vi "ReadLeftShiftRegister.vi"(1 "reference":refnum<vi>) -> (0 "LeftShiftRegister":T4)   [LabVIEW 2013]
uses:
  <vilib>/Utility/miscctls.llb/LVBoundsTypeDef.ctl
  <vilib>/Utility/miscctls.llb/LVPositionTypeDef.ctl
  <vilib>/Utility/miscctls.llb/LVRectTypeDef.ctl
panel:
  out "error out 17":errorcluster
  out "error out 16":errorcluster
  out "error out 15":errorcluster
  out "error out 14":errorcluster
  out "error out 13":errorcluster
  out "error out 12":errorcluster
  out "error out 11":errorcluster
  out "error out 10":errorcluster
  out "error out 9":errorcluster
  out "error out 8":errorcluster
  out "error out 7":errorcluster
  out "error out 6":errorcluster
  out "error out 5":errorcluster
  out "error out 4":errorcluster
  out "error out 3":errorcluster
  out "error out 2":errorcluster
  out "error out":errorcluster
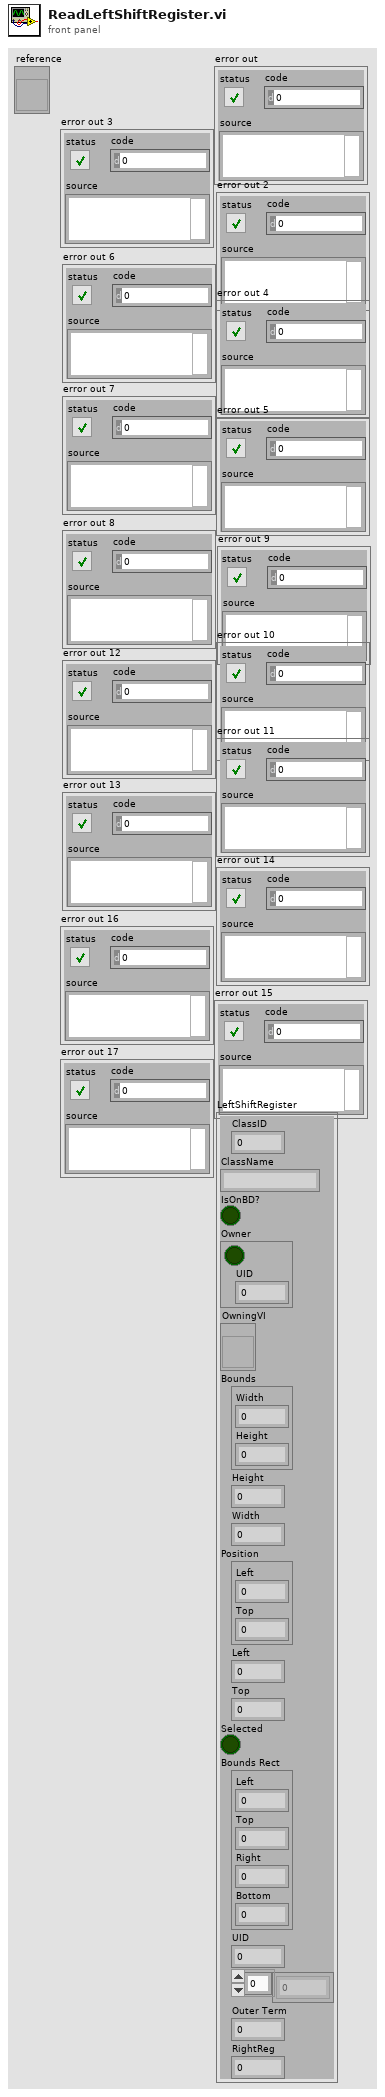
[diagram p1: front panel]
types:
  T1 = typedef "LVBoundsTypeDef.ctl" = cluster{"Width":u32, "Height":u32}
  T2 = typedef "LVPositionTypeDef.ctl" = cluster{"Left":i32, "Top":i32}
  T3 = typedef "LVRectTypeDef.ctl" = cluster{"Left":i16, "Top":i16, "Right":i16, "Bottom":i16}
  T4 = cluster{"ClassID":u32, "ClassName":string, "IsOnBD?":bool, "Owner":cluster{bool, "UID":i32}, "OwningVI":refnum<vi>, "Bounds":T1, "Height":u32, "Width":u32, "Position":T2, "Left":i32, "Top":i32, "Selected":bool, "Bounds Rect":T3, "UID":i32, "InsideTerms[]":i32[], "Outer Term":i32, "RightReg":i32}
  T5 = cluster{"ClassID":u32, "ClassName":string, "IsOnBD?":bool, "Cluster":cluster{bool, "UID":i32}, "OwningVI":refnum<vi>, "Bounds":T1, "Height":u32, "Width":u32, "Position":T2, "Left":i32, "Top":i32, "Selected":bool, "Bounds Rect":T3, "UID":i32, i32[], "UID":i32, "UID":i32}
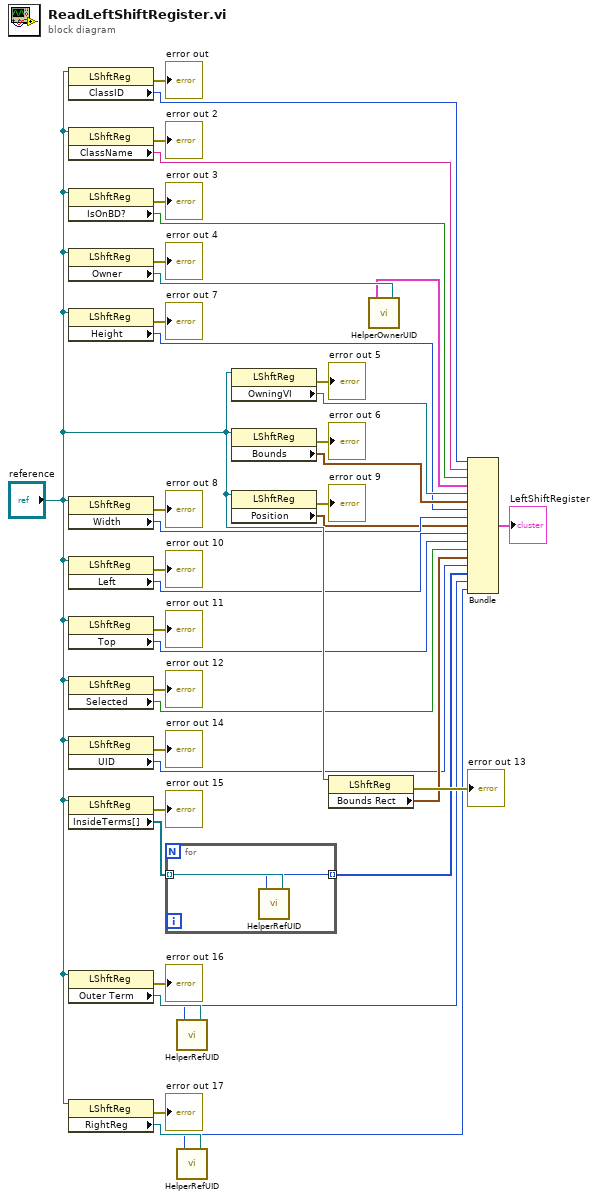
[diagram p0: block diagram]
diagram:
  n1 = property class="LShftReg"(reference="reference") -> (error out=→"error out":errorcluster, "ClassID"=w38:u32)  [unwired: 1 in, 1 out]
  n2 = property class="LShftReg"(reference="reference") -> (error out=→"error out 2":errorcluster, "ClassName"=w36:string)  [unwired: 1 in, 1 out]
  n3 = property class="LShftReg"(reference="reference") -> (error out=→"error out 3":errorcluster, "IsOnBD?"=w34:bool)  [unwired: 1 in, 1 out]
  n4 = property class="LShftReg"(reference="reference") -> (error out=→"error out 4":errorcluster, "Owner"=w32:refnum<vi>)  [unwired: 1 in, 1 out]
  n5 = property class="LShftReg"(reference="reference") -> (error out=→"error out 7":errorcluster, "Height"=w25:u32)  [unwired: 1 in, 1 out]
  n6 = property class="LShftReg"(reference="reference") -> (error out=→"error out 8":errorcluster, "Width"=w23:u32)  [unwired: 1 in, 1 out]
  n7 = property class="LShftReg"(reference="reference") -> (error out=→"error out 10":errorcluster, "Left"=w19:i32)  [unwired: 1 in, 1 out]
  n8 = property class="LShftReg"(reference="reference") -> (error out=→"error out 11":errorcluster, "Top"=w17:i32)  [unwired: 1 in, 1 out]
  n9 = property class="LShftReg"(reference="reference") -> (error out=→"error out 12":errorcluster, "Selected"=w15:bool)  [unwired: 1 in, 1 out]
  n10 = property class="LShftReg"(reference="reference") -> (error out=→"error out 14":errorcluster, "UID"=w11:i32)  [unwired: 1 in, 1 out]
  n11 = property class="LShftReg"(reference="reference") -> (error out=→"error out 15":errorcluster, "InsideTerms[]"=w9:refnum<vi>[])  [unwired: 1 in, 1 out]
  n12 = property class="LShftReg"(reference="reference") -> (error out=→"error out 16":errorcluster, "Outer Term"=w6:refnum<vi>)  [unwired: 1 in, 1 out]
  n13 = property class="LShftReg"(reference="reference") -> (error out=→"error out 17":errorcluster, "RightReg"=w3:refnum<vi>)  [unwired: 1 in, 1 out]
  n14 = for {
    tunnel: w9 -> [w42] mode=indexing
    tunnel: [w41] -> w8 mode=indexing
    n15 = call "HelperRefUID.vi"("Text in"=w42) -> ("UID"=w41:i32)
  }
  n16 = call "HelperRefUID.vi"("Text in"=w6) -> ("UID"=w5:i32)
  n17 = call "HelperRefUID.vi"("Text in"=w3) -> ("UID"=w2:i32)
  n18 = property class="LShftReg"(reference="reference") -> (error out=→"error out 5":errorcluster, "OwningVI"=w29:refnum<vi>)  [unwired: 1 in, 1 out]
  n19 = property class="LShftReg"(reference="reference") -> (error out=→"error out 6":errorcluster, "Bounds"=w27:T1)  [unwired: 1 in, 1 out]
  n20 = property class="LShftReg"(reference="reference") -> (error out=→"error out 9":errorcluster, "Position"=w21:T2)  [unwired: 1 in, 1 out]
  n21 = property class="LShftReg"(reference="reference") -> (error out=→"error out 13":errorcluster, "Bounds Rect"=w13:T3)  [unwired: 1 in, 1 out]
  n22 = call "HelperOwnerUID.vi"("Generic in"=w32) -> ("Cluster"=w31:cluster{bool, "UID":i32})
  n23 = Bundle("ClassID"=w38, "ClassName"=w36, "IsOnBD?"=w34, "Cluster"=w31, "OwningVI"=w29, "Bounds"=w27, "Height"=w25, "Width"=w23, "Position"=w21, "Left"=w19, "Top"=w17, "Selected"=w15, "Bounds Rect"=w13, "UID"=w11, w8, "UID"=w5, "UID"=w2) -> (→"LeftShiftRegister":T5)  [unwired: 1 in]
